vi "ADCDataRecorder.vi"() -> ()   [LabVIEW 2021]
uses:
  <vilib>/Utility/error.llb/DialogType.ctl
  <vilib>/DAQmx/read.llb/DAQmx Read (Analog 2D DBL NChan NSamp).vi
  <vilib>/DAQmx/create/channels.llb/DAQmx Create Channel (AI-Voltage-Basic).vi
  <vilib>/DAQmx/configure/timing.llb/DAQmx Timing (Sample Clock).vi
  <vilib>/DAQmx/miscellaneous.llb/DAQmx Fill In Error Info.vi
  <resource>/objmgr/daqmx.rc
panel:
  in  "Clear":bool
  out "NChannels":i32
  out "Time":string
  out "Parameter Text":string
  in  "Try to Read Parameters":bool
  in  "Parameters to Save":string="ParameterSweeper\nSetting\n"
  in  "Amplifier / V":dbl=1.0 format="%#_6p"
  in  "Sense / 10 V":dbl=10.0 format="%#_6p"
  in  "Save To File":bool
  in  "Header Text for Data Files":string
  in  "File Name to Save (auto incremented)":path
  in  "Measure":bool
  in  "Physical Channels":tag="Dev1/ai0:1"
  in  "Rate (Hz)":dbl=100.0 format="%#_3p"
  out "Waveform":dbl[][](graph)=[[2.1879798361445096e-13, 2.1815845753179685e-13, 2.1943750969771527e-13, 2.1943750969771527e-13, 2.1751893144975284e-13, 2.1879798361445096e-13, 2.1815845753179685e-13, 2.1943750969771527e-13, 2.1879798361445096e-13, 2.1815845753179685e-13, 2.1815845753179685e-13, 2.1879798361445096e-13, 2.1815845753179685e-13, 2.1815845753179685e-13, 2.1815845753179685e-13, 2.1815845753179685e-13, 2.1879798361445096e-13, 2.2007703578158964e-13, 2.1815845753179685e-13, 2.1943750969771527e-13, 2.1943750969771527e-13, 2.1879798361445096e-13, 2.1815845753179685e-13, 2.1815845753179685e-13, 2.1815845753179685e-13, 2.1879798361445096e-13, 2.1879798361445096e-13, 2.1879798361445096e-13, 2.1815845753179685e-13, 2.1815845753179685e-13, 2.1943750969771527e-13, 2.1879798361445096e-13, 2.1879798361445096e-13, 2.1879798361445096e-13, 2.1879798361445096e-13, 2.2007703578158964e-13, 2.1943750969771527e-13, 2.2007703578158964e-13, 2.1879798361445096e-13, 2.1815845753179685e-13, 2.1943750969771527e-13, 2.1943750969771527e-13, 2.2007703578158964e-13, 2.2071656186607413e-13, 2.1879798361445096e-13, 2.1879798361445096e-13, 2.1815845753179685e-13, 2.1879798361445096e-13, 2.1879798361445096e-13, 2.1751893144975284e-13, 2.1879798361445096e-13, 2.1815845753179685e-13, 2.1879798361445096e-13, 2.1879798361445096e-13, 2.1815845753179685e-13, 2.1879798361445096e-13, 2.1815845753179685e-13, 2.1751893144975284e-13, 2.1879798361445096e-13, 2.1943750969771527e-13, 2.1879798361445096e-13, 2.2007703578158964e-13, 2.1815845753179685e-13, 2.1879798361445096e-13, 2.1751893144975284e-13, 2.1815845753179685e-13, 2.1815845753179685e-13, 2.1879798361445096e-13, 2.1815845753179685e-13, 2.1879798361445096e-13, 2.1879798361445096e-13, 2.1879798361445096e-13, 2.1943750969771527e-13, 2.1943750969771527e-13, 2.1815845753179685e-13, 2.1815845753179685e-13, 2.1879798361445096e-13, 2.1943750969771527e-13, 2.1815845753179685e-13, 2.1943750969771527e-13, 2.1943750969771527e-13, 2.1879798361445096e-13, 2.1943750969771527e-13, 2.1879798361445096e-13, 2.1879798361445096e-13, 2.1879798361445096e-13, 2.1943750969771527e-13, 2.1943750969771527e-13, 2.1943750969771527e-13, 2.1879798361445096e-13, 2.1815845753179685e-13, 2.1879798361445096e-13, 2.1815845753179685e-13, 2.1815845753179685e-13, 2.1879798361445096e-13, 2.1879798361445096e-13, 2.1815845753179685e-13, 2.1879798361445096e-13, 2.1879798361445096e-13, 2.1815845753179685e-13], [3.774866786703138e-13, 3.7684717344553435e-13, 3.774866786703138e-13, 3.774866786703138e-13, 3.755681629996769e-13, 3.755681629996769e-13, 3.7684717344553435e-13, 3.7684717344553435e-13, 3.7684717344553435e-13, 3.762076682219888e-13, 3.755681629996769e-13, 3.755681629996769e-13, 3.7684717344553435e-13, 3.762076682219888e-13, 3.774866786703138e-13, 3.755681629996769e-13, 3.762076682219888e-13, 3.7684717344553435e-13, 3.762076682219888e-13, 3.755681629996769e-13, 3.762076682219888e-13, 3.7684717344553435e-13, 3.749286577785989e-13, 3.762076682219888e-13, 3.7684717344553435e-13, 3.762076682219888e-13, 3.762076682219888e-13, 3.7684717344553435e-13, 3.7684717344553435e-13, 3.7684717344553435e-13, 3.774866786703138e-13, 3.774866786703138e-13, 3.7684717344553435e-13, 3.762076682219888e-13, 3.762076682219888e-13, 3.7684717344553435e-13, 3.762076682219888e-13, 3.762076682219888e-13, 3.774866786703138e-13, 3.774866786703138e-13, 3.7684717344553435e-13, 3.7684717344553435e-13, 3.7684717344553435e-13, 3.7684717344553435e-13, 3.7684717344553435e-13, 3.774866786703138e-13, 3.762076682219888e-13, 3.755681629996769e-13, 3.7684717344553435e-13, 3.762076682219888e-13, 3.7684717344553435e-13, 3.755681629996769e-13, 3.762076682219888e-13, 3.7684717344553435e-13, 3.781261838963268e-13, 3.762076682219888e-13, 3.762076682219888e-13, 3.749286577785989e-13, 3.7684717344553435e-13, 3.7684717344553435e-13, 3.762076682219888e-13, 3.7684717344553435e-13, 3.755681629996769e-13, 3.7684717344553435e-13, 3.7684717344553435e-13, 3.755681629996769e-13, 3.762076682219888e-13, 3.7684717344553435e-13, 3.762076682219888e-13, 3.7684717344553435e-13, 3.762076682219888e-13, 3.7684717344553435e-13, 3.762076682219888e-13, 3.762076682219888e-13, 3.762076682219888e-13, 3.755681629996769e-13, 3.7684717344553435e-13, 3.7684717344553435e-13, 3.762076682219888e-13, 3.7684717344553435e-13, 3.774866786703138e-13, 3.7684717344553435e-13, 3.762076682219888e-13, 3.755681629996769e-13, 3.7684717344553435e-13, 3.762076682219888e-13, 3.762076682219888e-13, 3.762076682219888e-13, 3.7684717344553435e-13, 3.7684717344553435e-13, 3.762076682219888e-13, 3.762076682219888e-13, 3.762076682219888e-13, 3.762076682219888e-13, 3.762076682219888e-13, 3.781261838963268e-13, 3.7684717344553435e-13, 3.762076682219888e-13, 3.762076682219888e-13, 3.755681629996769e-13], [1.5212145151884067e-13, 1.5340108490468218e-13, 1.5276126821111775e-13, 1.5276126821111775e-13, 1.5276126821111775e-13, 1.5340108490468218e-13, 1.5276126821111775e-13, 1.5276126821111775e-13, 1.5212145151884067e-13, 1.5276126821111775e-13, 1.5276126821111775e-13, 1.5276126821111775e-13, 1.5276126821111775e-13, 1.5212145151884067e-13, 1.5276126821111775e-13, 1.5276126821111775e-13, 1.5340108490468218e-13, 1.5276126821111775e-13, 1.5212145151884067e-13, 1.5340108490468218e-13, 1.5212145151884067e-13, 1.5212145151884067e-13, 1.5276126821111775e-13, 1.5212145151884067e-13, 1.5276126821111775e-13, 1.5340108490468218e-13, 1.5276126821111775e-13, 1.5276126821111775e-13, 1.5340108490468218e-13, 1.5276126821111775e-13, 1.5276126821111775e-13, 1.5276126821111775e-13, 1.5212145151884067e-13, 1.5276126821111775e-13, 1.5212145151884067e-13, 1.5212145151884067e-13, 1.5276126821111775e-13, 1.5212145151884067e-13, 1.5276126821111775e-13, 1.5276126821111775e-13, 1.5276126821111775e-13, 1.5276126821111775e-13, 1.5276126821111775e-13, 1.5276126821111775e-13, 1.5276126821111775e-13, 1.5276126821111775e-13, 1.5340108490468218e-13, 1.5212145151884067e-13, 1.5276126821111775e-13, 1.5276126821111775e-13, 1.5212145151884067e-13, 1.5276126821111775e-13, 1.5212145151884067e-13, 1.5276126821111775e-13, 1.5276126821111775e-13, 1.5276126821111775e-13, 1.5340108490468218e-13, 1.5276126821111775e-13, 1.5212145151884067e-13, 1.5276126821111775e-13, 1.5212145151884067e-13, 1.5276126821111775e-13, 1.5276126821111775e-13, 1.5340108490468218e-13, 1.5340108490468218e-13, 1.5276126821111775e-13, 1.5276126821111775e-13, 1.5212145151884067e-13, 1.5276126821111775e-13, 1.5276126821111775e-13, 1.5276126821111775e-13, 1.5276126821111775e-13, 1.5276126821111775e-13, 1.5276126821111775e-13, 1.5340108490468218e-13, 1.5212145151884067e-13, 1.5212145151884067e-13, 1.5276126821111775e-13, 1.5276126821111775e-13, 1.5276126821111775e-13, 1.5276126821111775e-13, 1.5276126821111775e-13, 1.5212145151884067e-13, 1.5276126821111775e-13, 1.5276126821111775e-13, 1.5276126821111775e-13, 1.5276126821111775e-13, 1.5276126821111775e-13, 1.5276126821111775e-13, 1.5212145151884067e-13, 1.5212145151884067e-13, 1.5276126821111775e-13, 1.5276126821111775e-13, 1.5276126821111775e-13, 1.5276126821111775e-13, 1.5212145151884067e-13, 1.5212145151884067e-13, 1.5212145151884067e-13, 1.5340108490468218e-13, 1.5276126821111775e-13]]
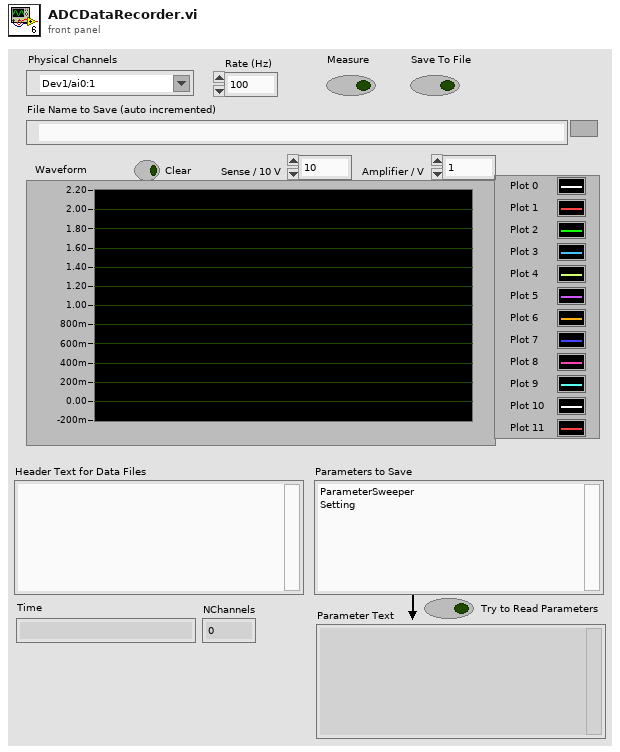
[diagram p1: front panel]
types:
  T1 = enum8{"Enabled", "Disabled", "Disabled and Grayed Out"}
  T2 = enum16{"open", "replace", "create", "open or create", "replace or create", "replace or create with confirmation"}
  T3 = typedef "DialogType.ctl" = u16
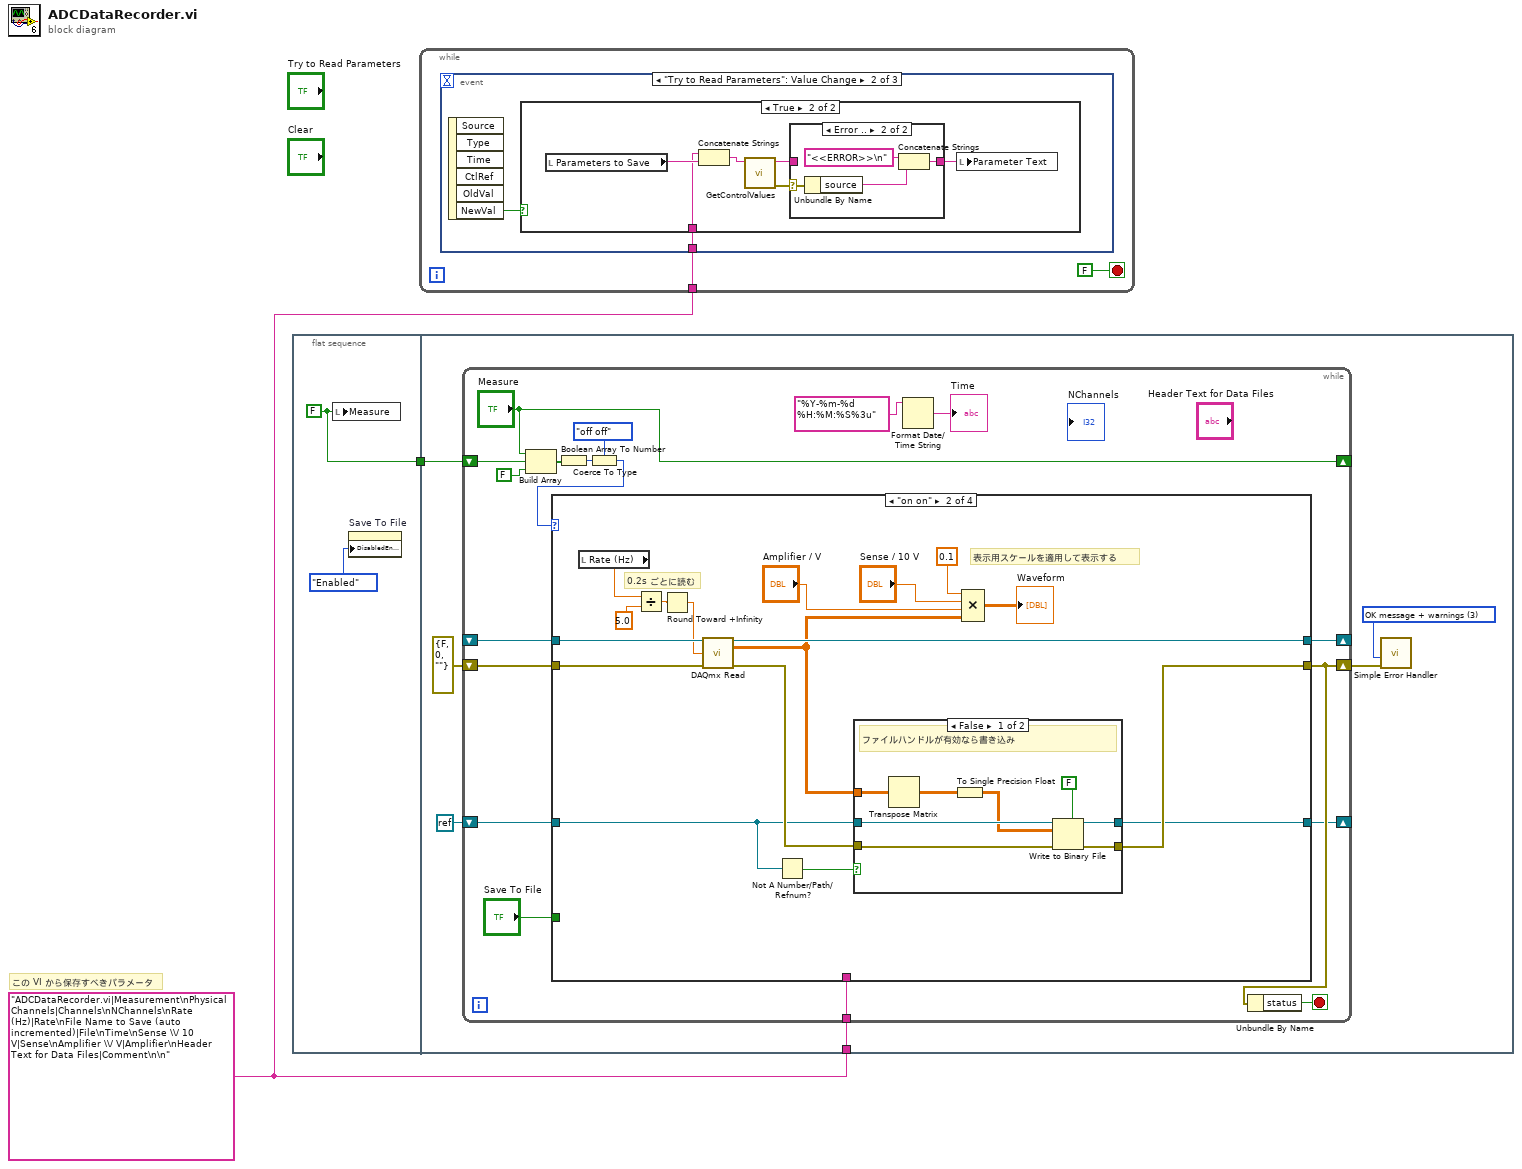
[diagram p0: block diagram]
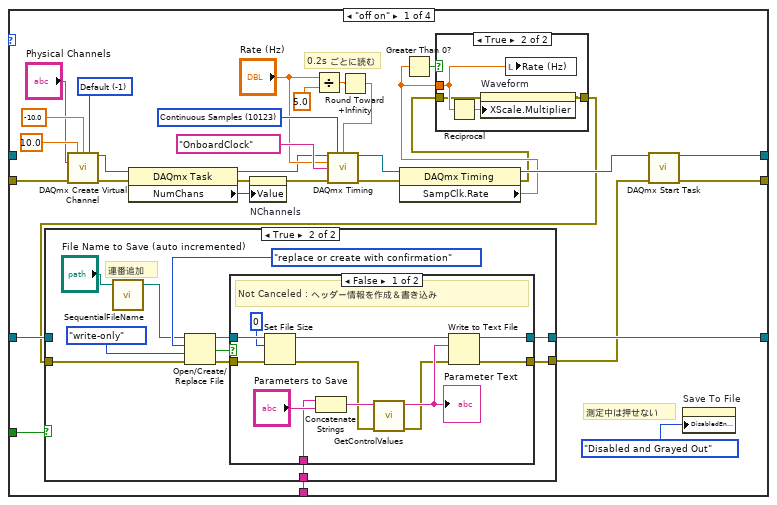
[diagram p2: hidden frame]
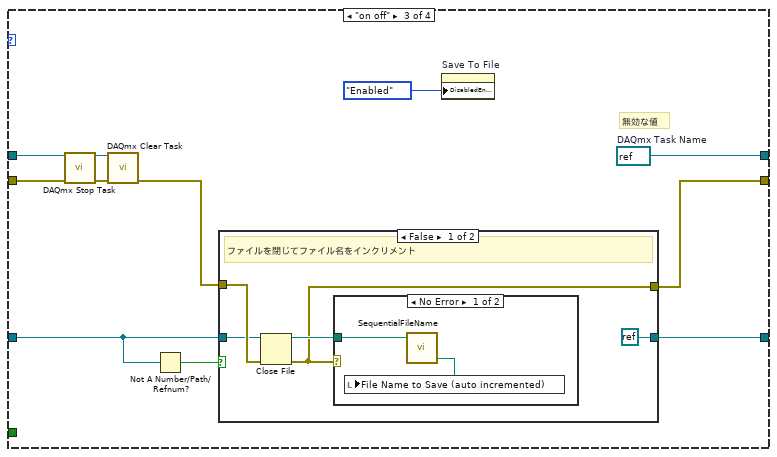
[diagram p7: hidden frame]
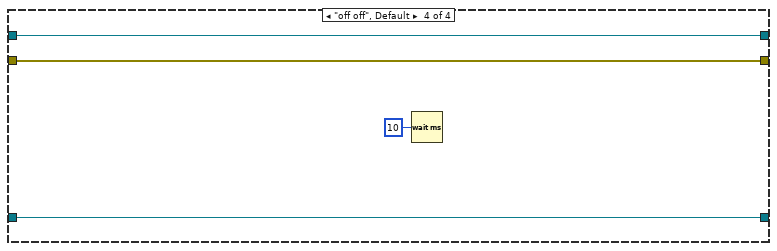
[diagram p10: hidden frame]
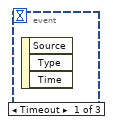
[diagram p11: hidden frame]
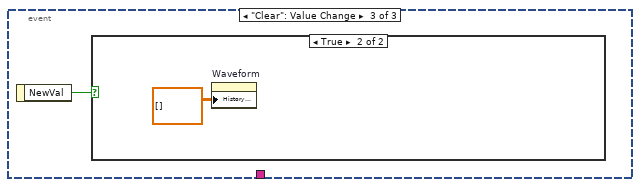
[diagram p14: hidden frame]
diagram:
  w1 = "ADCDataRecorder.vi|Measurement\nPhysical Channels|Channels\nNChannels\nRate (Hz)|Rate\nFile Name to Save (auto incremented)|File\nTime\nSense \\/ 10 V|Sense\nAmplifier \\/ V|Amplifier\nHeader Text for Data Files|Comment\n\n"
  # "この VI から保存すべきパラメータ"
  n1 = flat-sequence {
    tunnel: [w4] -> w2
    tunnel: w2 -> [w8]
    tunnel: w1 -> [w5]
    frame #0 {
      w4 = FALSE ("Measure")
      n2 = local write "Measure"(w4) -> ()
      n3 = property on="Save To File" class="Bool (strict)"("DisabledEnum"=T1."Enabled" ("Disabled")) -> ()  [unwired: 2 in, 2 out]
    }
    frame #1 {
      w10 = T3 3 items=["no dialog", "OK message", "continue or stop message", "OK message + warnings", "continue/stop + warnings"] ("type of dialog (OK msg:1)")
      n4 = while {
        shift-right: [w28] -> _
        shift-left: _ -> [w27]
        shift-right: [w25] -> w9
        shift-left: errorcluster {"status"=FALSE, "code"=0, "source"=""} ("error out") -> [w26]
        shift-right: ["Measure"] -> _
        shift-left: w8 -> [w17]
        shift-right: [w21] -> _
        shift-left: refnum<k0> refnum -> [w20]
        tunnel: w5 -> [w11]
        stop <- w24 stop-if-true
        n5 = Build Array("Measure", w17, FALSE ("element")) -> (w15:bool[])
        n6 = Boolean Array To Number(Boolean array=w15) -> (number=w14:u32)
        n7 = Coerce To Type(0:w14, 1:enum16{"off off", "off on", "on off", "on on"}."off off") -> (2:w22:enum16{"off off", "off on", "on off", "on on"})
        n8 = case shown="\"on on\"" w22 {
          tunnel: [w50 w109 w128 w143] -> w28
          tunnel: w27 -> [_ w107 w126 w143]
          tunnel: [w49 w105 w124 w142] -> w25
          tunnel: w26 -> [w44 w108 w127 w142]
          tunnel: [w48 w104 w121 w141] -> w21
          tunnel: w20 -> [w46 w102 w123 w141]
          tunnel: "Save To File" -> [w47 _ _ _]
          tunnel: w11 -> [w33 _ _ _]
          frame "off on" {
            w57 = 10123 items=["Finite Samples"=10178, "Continuous Samples"=10123, "Hardware Timed Single Point"=12522] ("sample mode")
            w58 = -1 items=["Default"=-1, "RSE"=10083, "Differential"=10106, "Pseudodifferential"=12529] ("output terminal configuration")
            # "測定中は押せない"
            # "0.2s ごとに読む"
            n9 = call-poly <vilib>:"DAQmx Create Virtual Channel.vi"("maximum value"=10.0, "minimum value"=-10.0, "input terminal configuration"=w58, "physical channels"="Physical Channels", "error in"=w44) -> ("task out"=w39:refnum<k21>, "error out"=w40:errorcluster)  [unwired: 9 in]
            n10 = property class="DAQmx Task"(reference=w39, error in=w40) -> (reference out=w38:refnum<k21>, error out=w36:errorcluster, "NumChans"=w34:u32)
            n11 = property on="NChannels" class="DigNum (strict)"(error in=w36, "Value"=w34) -> (error out=w35:errorcluster)  [unwired: 1 in, 1 out]
            n12 = Divide(x="Rate (Hz)", y=5.0) -> (x/y=w30:dbl)
            n13 = Round Toward +Infinity(x=w30) -> (ceil(x): smallest int >= x=w29:dbl)
            n14 = call-poly <vilib>:"DAQmx Timing.vi"("task/channels in"=w38, "sample mode"=w57, "samples per channel"=w29, "rate"="Rate (Hz)", "source"=tag "OnboardClock", "error in"=w35) -> ("task out"=w53:refnum<k21>, "error out"=w54:errorcluster)  [unwired: 8 in]
            n15 = property class="DAQmx Timing"(reference=w53, error in=w54) -> (reference out=w55:refnum<k21>, error out=w32:errorcluster, "SampClk.Rate"=w37:dbl)
            n16 = Greater Than 0?(x=w37) -> (x > 0?=w45:bool)
            n17 = case shown="True" w45 {
              tunnel: w37 -> [_ w64]
              tunnel: w32 -> [w61 w63]
              tunnel: [w61 w62] -> w31
              frame False {
              }
              frame True {
                n18 = Reciprocal(x=w64) -> (1/x=w65:dbl)
                n19 = property on="Waveform" class="WFChart (strict)"(error in=w63, "XScale.Multiplier"=w65) -> (error out=w62:errorcluster)  [unwired: 1 in, 1 out]
                n20 = local write "Rate (Hz)"(w64) -> ()
              }
            }
            n21 = case shown="True" w47 {
              tunnel: [w66 w73] -> w48
              tunnel: w31 -> [w67 w72]
              tunnel: [w67 w71] -> w43
              tunnel: w46 -> [w66 _]
              tunnel: w33 -> [_ w68]
              frame False {
              }
              frame True {
                # "連番追加"
                n22 = call "SequentialFileName.vi"("File Name In"="File Name to Save (auto incremented)") -> ("File Name With Sequence"=w69:path)  [unwired: 3 in, 1 out]
                n23 = Open/Create/Replace File(file path (use dialog)=w69, error in=w72, operation (0:open)=T2."replace or create with confirmation" ("操作 (0:open)"), access (0:read/write)=enum16{"read/write", "read-only", "write-only"}."write-only" ("アクセス (0:read/write)")) -> (refnum out=w78:refnum<file>, cancelled=w70:bool, error out=w75:errorcluster)  [unwired: 2 in]
                n24 = case shown="False" w70 {
                  tunnel: w78 -> [w90 w92]
                  tunnel: w75 -> [w84 w91]
                  tunnel: [w87 w92] -> w73
                  tunnel: [w86 w91] -> w71
                  tunnel: w68 -> [w82 _]
                  frame False {
                    # "Not Canceled : ヘッダー情報を作成＆書き込み"
                    n25 = Set File Size(4:w84, 6:i64 0 ("サイズ (バイト)"), 7:w90) -> (0:w81:errorcluster, 3:w89:refnum<file>)
                    n26 = Concatenate Strings(w82, "Parameters to Save") -> (w83:string)
                    n27 = call "GetControlValues.vi"("error in"=w81, "ControlList"=w83) -> ("error out"=w79:errorcluster, "Control Values"=w80:string)  [unwired: 8 in]
                    "Parameter Text" <- w80
                    n28 = Write to Text File(file (use dialog)=w89, text=w80, error in=w79) -> (refnum out=w87:refnum<file>, error out=w86:errorcluster)  [unwired: 1 in, 1 out]
                  }
                  frame True {
                    # "Canceled"
                  }
                }
              }
            }
            n29 = call <vilib>:"DAQmx Start Task.vi"("task/channels in"=w55, "error in"=w43) -> ("task out"=w50:refnum<k21>, "error out"=w49:errorcluster)  [unwired: 12 in]
            n30 = property on="Save To File" class="Bool (strict)"("DisabledEnum"=T1."Disabled and Grayed Out" ("Disabled")) -> ()  [unwired: 2 in, 2 out]
          }
          frame "on on" {
            # "0.2s ごとに読む"
            # "表示用スケールを適用して表示する"
            n31 = local read "Rate (Hz)"() -> (w94:dbl)
            n32 = Divide(x=w94, y=5.0) -> (x/y=w95:dbl)
            n33 = Round Toward +Infinity(x=w95) -> (ceil(x): smallest int >= x=w93:dbl)
            n34 = call-poly <vilib>:"DAQmx Read.vi"("task/channels in"=w107, "number of samples per channel"=w93, "error in"=w108) -> ("task out"=w109:refnum<k21>, "data"=w97:dbl[][], "error out"=w106:errorcluster)  [unwired: 10 in]
            n35 = Not A Number/Path/Refnum?(number/path/refnum=w102) -> (NaN/Path/Refnum?=w103:bool)
            n36 = case shown="False" w103 {
              tunnel: w106 -> [w116 w119]
              tunnel: [w115 w119] -> w105
              tunnel: w102 -> [w114 w118]
              tunnel: [w113 w118] -> w104
              tunnel: w97 -> [w111 _]
              frame False {
                # "ファイルハンドルが有効なら書き込み"
                n37 = Transpose Matrix(1:w111) -> (0:w110:dbl[][])
                n38 = To Single Precision Float(number=w110) -> (single precision float=w112:sgl[][])
                n39 = Write to Binary File(file (use dialog)=w114, data=w112, error in=w116, 5:FALSE ("配列または文字列サイズを先頭に追加? (T)")) -> (refnum out=w113:refnum<file>, error out=w115:errorcluster)  [unwired: 2 in, 1 out]
              }
              frame True {
              }
            }
            n40 = Compound Arithmetic op=MULTIPLY(0.1 ("value"), "Sense / 10 V", "Amplifier / V", w97) -> (→"Waveform":dbl[][])
          }
          frame "on off" {
            w128 = refnum<k21> refnum  # DAQmx Task Name
            # "無効な値"
            n41 = call <vilib>:"DAQmx Stop Task.vi"("task/channels in"=w126, "error in"=w127) -> ("task out"=w129:refnum<k21>, "error out"=w130:errorcluster)  [unwired: 12 in]
            n42 = call <vilib>:"DAQmx Clear Task.vi"("task in"=w129, "error in"=w130) -> ("error out"=w125:errorcluster)  [unwired: 13 in]
            n43 = Not A Number/Path/Refnum?(number/path/refnum=w123) -> (NaN/Path/Refnum?=w122:bool)
            n44 = case shown="False" w122 {
              tunnel: w125 -> [w134 w139]
              tunnel: [w133 w139] -> w124
              tunnel: w123 -> [w132 w138]
              tunnel: [refnum<k0> refnum w138] -> w121
              frame False {
                # "ファイルを閉じてファイル名をインクリメント"
                n45 = Close File(refnum=w132, error in=w134) -> (path=w135:path, error out=w133:errorcluster)
                n46 = case shown="No Error" w133 {
                  tunnel: w135 -> [w137 _]
                  frame No Error {
                    n47 = call "SequentialFileName.vi"("File Name In"=w137) -> ("Next File Name"=w136:path)  [unwired: 3 in, 1 out]
                    n48 = local write "File Name to Save (auto incremented)"(w136) -> ()
                  }
                  frame Error {
                  }
                }
              }
              frame True {
              }
            }
            n49 = property on="Save To File" class="Bool (strict)"("DisabledEnum"=T1."Enabled" ("Disabled")) -> ()  [unwired: 2 in, 2 out]
          }
          frame "off off", Default {
            n50 = Wait (ms)(milliseconds to wait=u32 10) -> ()  [unwired: 1 out]
          }
        }
        n51 = Format Date/Time String(time format string (%c)="%Y-%m-%d %H:%M:%S%3u" ("時間形式文字列 (%c)")) -> (date/time string=→"Time":string)  [unwired: 2 in]
        n52 = Unbundle By Name(w25) -> ("status"=w24:bool)
      }
      n53 = call <vilib>:"Simple Error Handler.vi"("type of dialog (OK msg:1)"=w10, "error in (no error)"=w9) -> ()  [unwired: 3 in, 5 out]
    }
  }
  n54 = while {
    tunnel: w1 -> [w144]
    stop <- FALSE stop-if-true
    n55 = event shown="[1] \"Try to Read Parameters\": Value Change" {
      selector: _ -> [_ _ _]
      dyn-events: _ -> [_ _ _]
      timeout: _ -> [_ _ _]
      tunnel: w144 -> [_ w146 _]
      event Timeout {
        n56 = event-data() -> ()  [unwired: 1 in, 3 out]
      }
      event "Try to Read Parameters": Value Change {
        n57 = event-data() -> ("NewVal"=w147:bool)  [unwired: 1 in, 5 out]
        n58 = case shown="True" w147 {
          tunnel: w146 -> [_ w148]
          frame False {
          }
          frame True {
            n59 = local read "Parameters to Save"() -> (w150:string)
            n60 = Concatenate Strings(w148, w150) -> (w149:string)
            n61 = call "GetControlValues.vi"("ControlList"=w149) -> ("error out"=w153:errorcluster, "Control Values"=w152:string)  [unwired: 9 in]
            n62 = case shown="Error .." w153 {
              selector: w153 -> [_ w158]
              tunnel: w152 -> [w154 _]
              tunnel: [w154 w157] -> w151
              frame No Error {
              }
              frame Error {
                n63 = Unbundle By Name(w158) -> ("source"=w156:string)
                n64 = Concatenate Strings("<<ERROR>>\n", w156) -> (w157:string)
              }
            }
            n65 = local write "Parameter Text"(w151) -> ()
          }
        }
      }
      event "Clear": Value Change {
        n66 = event-data() -> ("NewVal"=w159:bool)  [unwired: 1 in]
        n67 = case shown="True" w159 {
          frame False {
          }
          frame True {
            n68 = property on="Waveform" class="WFChart (strict)"("History Data"=dbl[][] []) -> ()  [unwired: 2 in, 2 out]
          }
        }
      }
    }
  }
